vi "Read gRPC Configuration File.vi"(8 "error in":errorcluster) -> (0 "error out":errorcluster, 1 "Manager Server Address":string, 2 "Plugin Server Address":string, 3 "Server Certificate File (.crt)":path, 4 "Local Manager Address":string, 5 "Server Key File (.key)":path)   [LabVIEW 2021, in "gRPC Configuration File.lvlib"]
uses:
  gRPC Configuration File.lvlib
  <vilib>/Utility/config.llb/Read Key (String).vi
  <vilib>/Utility/config.llb/Read Key (I32).vi
  <vilib>/Utility/config.llb/Read Key (Path).vi
  <vilib>/Utility/config.llb/NI_LVConfig.lvlib
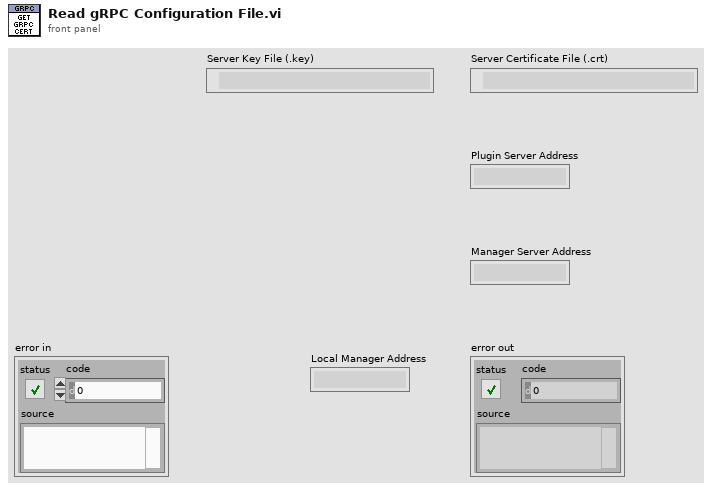
[diagram p1: front panel]
types:
  T1 = typedef "NI_LVConfig.lvlib/Config Data RefNum.ctl" = refnum<k1>
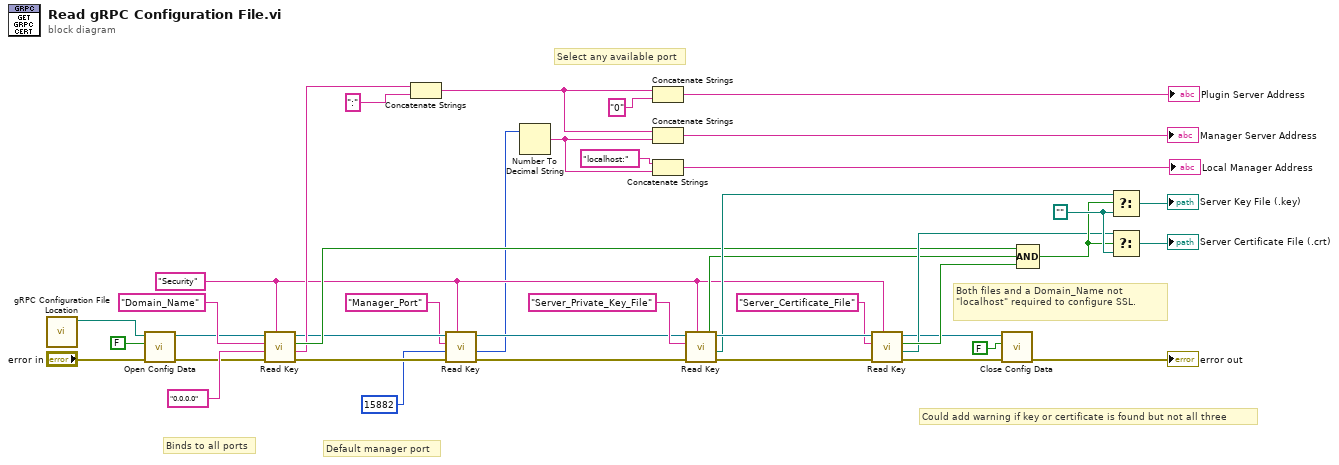
[diagram p0: block diagram]
diagram:
  w34 = path ""
  w10 = "Security" ("Section")
  # "Could add warning if key or certificate is found but not all three"
  # "Select any available port"
  # "Default manager port"
  # "Binds to all ports"
  # "Both files and a Domain_Name not \"localhost\" required to configure SSL."
  n1 = call "gRPC Configuration File Location.vi"() -> ("configuration file path"=w27:path)  [unwired: 11 in]
  n2 = call <vilib>:"Open Config Data.vi"("error in (no error)"="error in", "create file if necessary (T)"=FALSE, "configuration file path"=w27) -> ("error out"=w5:errorcluster, "refnum"=w4:T1)  [unwired: 6 in, 1 out]
  n3 = call-poly <vilib>:"Read Key.vi"("section"=w10, "error in (no error)"=w5, "default value"="0.0.0.0", "key"="Domain_Name", "refnum"=w4) -> ("error out"=w13:errorcluster, "value"=w19:string, "found?"=w20:bool, "refnum out"=w14:T1)  [unwired: 3 in]
  n4 = Concatenate Strings(w19, ":" ("string")) -> (w18:string)
  n5 = call-poly <vilib>:"Read Key.vi"("section"=w10, "error in (no error)"=w13, "default value"=15882, "key"="Manager_Port", "refnum"=w14) -> ("error out"=w11:errorcluster, "value"=w7:i32, "refnum out"=w12:T1)  [unwired: 3 in, 1 out]
  n6 = Number To Decimal String(number=w7) -> (decimal integer string=w3:string)  [unwired: 1 in]
  n7 = Concatenate Strings(w18, "0" ("string")) -> (→"Plugin Server Address":string)
  n8 = Concatenate Strings(w18, w3) -> (→"Manager Server Address":string)
  n9 = Concatenate Strings("localhost:" ("string"), w3) -> (→"Local Manager Address":string)
  n10 = call-poly <vilib>:"Read Key.vi"("section"=w10, "error in (no error)"=w11, "key"="Server_Private_Key_File", "refnum"=w12) -> ("error out"=w37:errorcluster, "value"=w31:path, "found?"=w26:bool, "refnum out"=w35:T1)  [unwired: 4 in]
  n11 = call-poly <vilib>:"Read Key.vi"("section"=w10, "error in (no error)"=w37, "key"="Server_Certificate_File", "refnum"=w35) -> ("error out"=w21:errorcluster, "value"=w30:path, "found?"=w33:bool, "refnum out"=w22:T1)  [unwired: 4 in]
  n12 = call <vilib>:"Close Config Data.vi"("error in (no error)"=w21, "write file if changed (T)"=FALSE, "refnum"=w22) -> ("error out"=→"error out":errorcluster)  [unwired: 7 in, 1 out]
  n13 = Compound Arithmetic op=AND(w20, w26, w33) -> (w32:bool)
  n14 = Select(t=w31, s=w32, f=w34) -> (s? t:f=→"Server Key File (.key)":path)
  n15 = Select(t=w30, s=w32, f=w34) -> (s? t:f=→"Server Certificate File (.crt)":path)
